vi "Status.vi"(0 "Serial Controller in":refnum<class "Serial Controller.lvclass">, 11 "error in (no error)":errorcluster) -> (3 "Hi Resolution":bool, 4 "Serial Controller out":refnum<class "Serial Controller.lvclass">, 6 "Firmware Version":u16, 8 "Velocity mm/s":u16, 10 "Microsteps Per Pulse":u16, 12 "Multiplier msteps/mm":u16, 13 "Divisor msteps/mm":u16, 14 "Adjusted Pulse Speed":u16, 15 "error out":errorcluster)   [LabVIEW 2014, in "Serial Controller.lvclass"]
uses:
  Serial Controller.lvclass
  Serial Controller.lvclass/Serial Controller.ctl
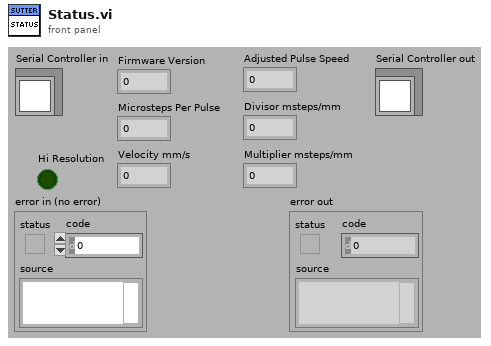
[diagram p1: front panel]
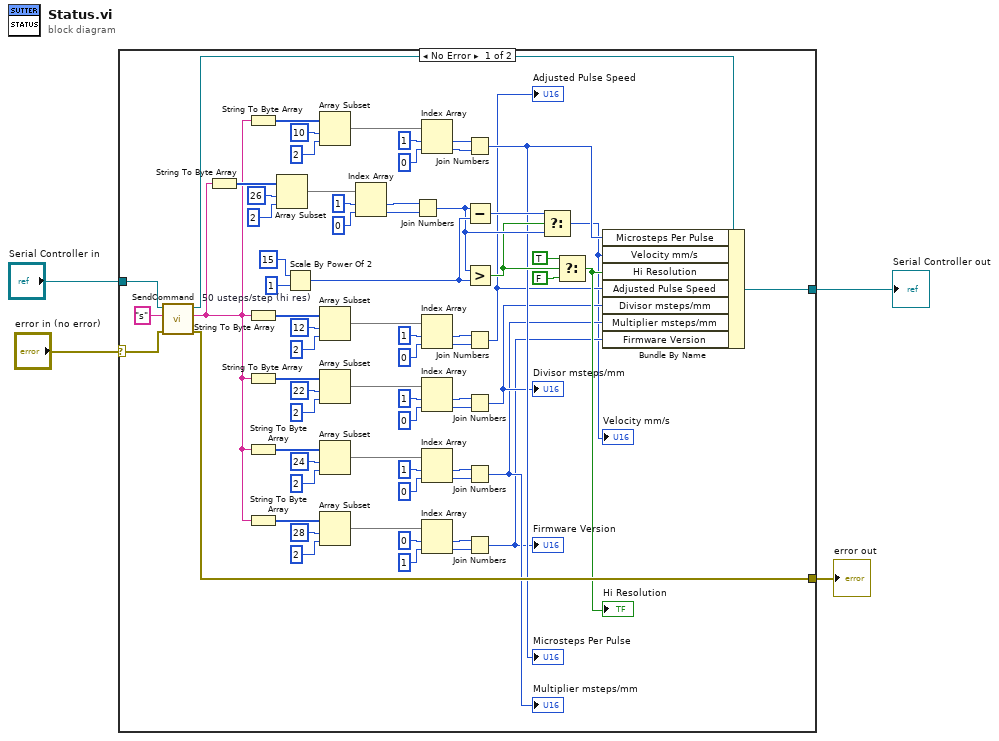
[diagram p0: block diagram]
diagram:
  n1 = case shown="No Error" "error in (no error)" {
    selector: "error in (no error)" -> [w65 w76]
    tunnel: [w64 w76] -> w3
    tunnel: [w6 w75] -> w1
    tunnel: "Serial Controller in" -> [w66 w75]
    frame No Error {
      n2 = call-dynamic "SendCommand.vi"("error in (no error)"=w65, "command"="s", "Serial Controller in"=w66) -> ("error out"=w64:errorcluster, "Returned"=w9:string, "Serial Controller out"=w30:refnum<class "Serial Controller.lvclass">)  [unwired: 6 in]
      n3 = String To Byte Array(string=w9) -> (unsigned byte array=w54:u8[])
      n4 = String To Byte Array(string=w9) -> (unsigned byte array=w62:u8[])
      n5 = String To Byte Array(string=w9) -> (unsigned byte array=w38:u8[])
      n6 = String To Byte Array(string=w9) -> (unsigned byte array=w26:u8[])
      n7 = String To Byte Array(string=w9) -> (unsigned byte array=w17:u8[])
      n8 = String To Byte Array(string=w9) -> (unsigned byte array=w74:u8[])
      n9 = Array Subset(array=w54, index=26, length=2) -> (w51:u8[])
      n10 = Scale By Power Of 2 "50 usteps/step (hi res)"(n=i16 15, x=u16 1) -> (x*2^n=w43:u16)
      n11 = Array Subset(array=w62, index=10, length=2) -> (w59:u8[])
      n12 = Array Subset(array=w38, index=12, length=2) -> (w35:u8[])
      n13 = Array Subset(array=w26, index=22, length=2) -> (w23:u8[])
      n14 = Array Subset(array=w17, index=24, length=2) -> (w14:u8[])
      n15 = Array Subset(array=w74, index=28, length=2) -> (w71:u8[])
      n16 = Index Array(array=w51, index #1=1 ("index"), index #2=0 ("index")) -> (element #1=w48:u8, element #2=w47:u8)
      n17 = Join Numbers(hi=w48, lo=w47) -> ((hi.lo)=w42:u16)
      n18 = Index Array(array=w59, index #1=1 ("index"), index #2=0 ("index")) -> (element #1=w56:u8, element #2=w55:u8)
      n19 = Index Array(array=w35, index #1=1 ("index"), index #2=0 ("index")) -> (element #1=w32:u8, element #2=w31:u8)
      n20 = Index Array(array=w23, index #1=1 ("index"), index #2=0 ("index")) -> (element #1=w20:u8, element #2=w19:u8)
      n21 = Index Array(array=w14, index #1=1 ("index"), index #2=0 ("index")) -> (element #1=w11:u8, element #2=w10:u8)
      n22 = Index Array(array=w71, index #1=0 ("index"), index #2=1 ("index")) -> (element #1=w68:u8, element #2=w67:u8)
      n23 = Join Numbers(hi=w56, lo=w55) -> ((hi.lo)=w29:u16)
      "Microsteps Per Pulse" <- w29
      n24 = Subtract(x=w42, y=w43) -> (x-y=w44:u16)
      n25 = Greater?(x=w42, y=w43) -> (0:w41:bool)
      n26 = Join Numbers(hi=w32, lo=w31) -> ((hi.lo)=w27:u16)
      "Adjusted Pulse Speed" <- w27
      n27 = Join Numbers(hi=w20, lo=w19) -> ((hi.lo)=w18:u16)
      "Divisor msteps/mm" <- w18
      n28 = Join Numbers(hi=w11, lo=w10) -> ((hi.lo)=w8:u16)
      "Multiplier msteps/mm" <- w8
      n29 = Join Numbers(hi=w68, lo=w67) -> ((hi.lo)=w7:u16)
      "Firmware Version" <- w7
      n30 = Select(t=w44, s=w41, f=w42) -> (s? t:f=w5:u16)
      "Velocity mm/s" <- w5
      n31 = Select(t=TRUE, s=w41, f=FALSE) -> (s? t:f=w28:bool)
      "Hi Resolution" <- w28
      n32 = Bundle By Name(cluster=w30, "Microsteps Per Pulse"=w29, "Velocity mm/s"=w5, "Hi Resolution"=w28, "Adjusted Pulse Speed"=w27, "Divisor msteps/mm"=w18, "Multiplier msteps/mm"=w8, "Firmware Version"=w7) -> (w6:refnum<class "Serial Controller.lvclass">)
    }
    frame Error {
    }
  }
  "error out" <- w3
  "Serial Controller out" <- w1
